vi "test email 2.vi"() -> ()   [LabVIEW 2016]
panel:
  out "error out":errorcluster
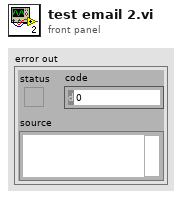
[diagram p1: front panel]
types:
  T1 = typedef "Array AE Data.ctl" = T2[]
  T2 = typedef "AE Data.ctl" = cluster{"Name":string, "Go?":bool, "Which batch?":enum16{"Anything", "First", "Second"}}
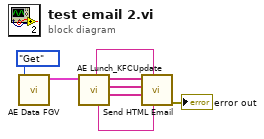
[diagram p0: block diagram]
diagram:
  n1 = call "AE Data FGV.vi"("Command"=enum16{"Initialize", "Update", "Get"}."Get") -> ("Array of AEs"=w7:T1)  [unwired: 9 in, 1 out]
  n2 = call "AE Lunch_KFCUpdate.vi"("Array of AEs"=w7) -> ("Not Going"=w4:string[], "Second Batch"=w5:string[], "First Batch"=w6:string[], "Second Batch Food"=w2:string, "First Batch Food"=w3:string)  [unwired: 6 in]
  n3 = call "Send HTML Email.vi"("Second Batch Food"=w2, "First Batch Food"=w3, "Not Going"=w4, "Second Batch"=w5, "First Batch"=w6) -> ("error out"=→"error out":errorcluster)  [unwired: 5 in, 1 out]
